vi "LVClass_CorrectionDataManager SetWaveFrontCorrectorPreferences.vi"(0 "CorrectionDataManager in":refnum<class "CorrectionDataManager.lvclass">, 9 "Wavefront Corrector State":T1[](array[typedef]), 11 "error in (no error)":errorcluster) -> (4 "CorrectionDataManager out":refnum<class "CorrectionDataManager.lvclass">, 8 "New data needed":bool, 15 "error out":errorcluster)   [LabVIEW 2020, in "CorrectionDataManager.lvclass"]
doc: "Wavefront corrector actuators preferences setter. The new preferences have to\nbe compliant with the Wavefront corrector specifications (read from\nconfiguration file).\n\n--------------------------------------------------------------------------------\n\n<B>corrdata_managerIn </B> : CorrDataManager object.\n<B>corrdata_managerOut </B> : CorrDataManager object.\n<B>min </B> : WavefrontCorrector preferences : lowest command value.\n<B>max </B> : WavefrontCorrector preferences : highest command value.\n<B>validity </B> : WavefrontCorrector preferences : status.\n<B>fixed_value </B> : WavefrontCorrector preferences : fixed positions.\n<B>ErrorIn </B> : Error\n<B>ErrorOut </B> : Error\n\n--------------------------------------------------------------------------------"
uses:
  CorrectionDataManager.lvclass
  Wavefront Corrector states - ONE.ctl
  CorrectionDataManager.lvclass/CorrectionDataManager.ctl
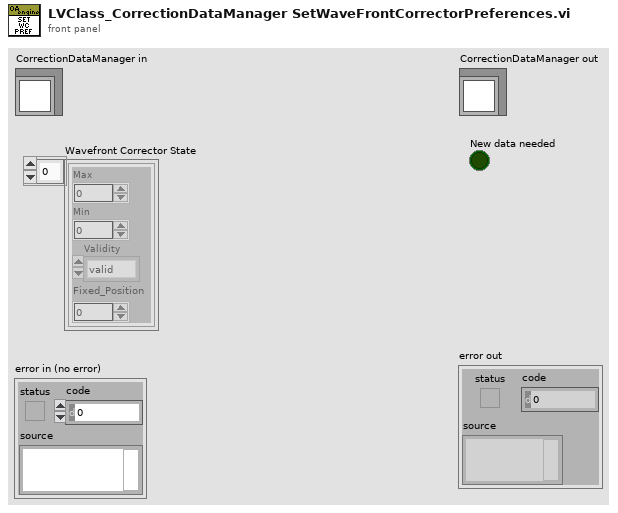
[diagram p1: front panel]
types:
  T1 = typedef "Wavefront Corrector states - ONE.ctl" = cluster{"Max":sgl, "Min":sgl, "Validity":enum16{"valid", "fixed", "invalid"}, "Fixed_Position":sgl}
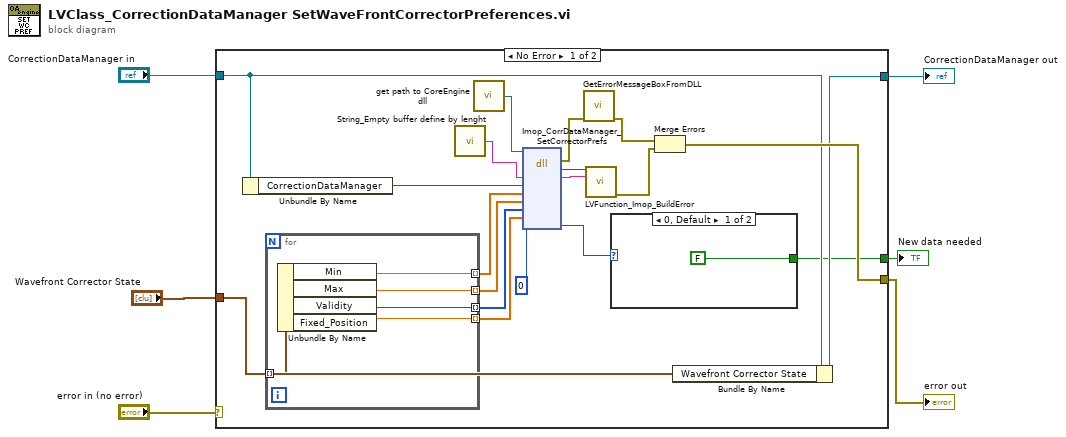
[diagram p0: block diagram]
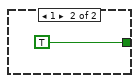
[diagram p2: hidden frame]
diagram:
  n1 = case shown="No Error" "error in (no error)" {
    selector: "error in (no error)" -> [_ w34]
    tunnel: [w23 w34] -> w3
    tunnel: [w11 w33] -> w4
    tunnel: "CorrectionDataManager in" -> [w12 w33]
    tunnel: "Wavefront Corrector State" -> [w10 _]
    tunnel: [w7 _] -> w1
    frame No Error {
      n2 = Unbundle By Name(w12) -> ("CorrectionDataManager"=w13:i32)
      n3 = for {
        tunnel: w10 -> [w32] mode=indexing
        tunnel: [w31] -> w15 mode=indexing
        tunnel: [w30] -> w14 mode=indexing
        tunnel: [w29] -> w17 mode=indexing
        tunnel: [w28] -> w16 mode=indexing
        n4 = Unbundle By Name(w32) -> ("Min"=w31:sgl, "Max"=w30:sgl, "Validity"=w29:enum16{"valid", "fixed", "invalid"}, "Fixed_Position"=w28:sgl)
      }
      n5 = call "String_Empty buffer define by lenght.vi"() -> ("Empty buffer"=w21:string)  [unwired: 1 in]
      n6 = call "get path to CoreEngine dll.vi"() -> ("path to c_interface_vc100.dll"=w22:path)  [unwired: 12 in, 3 out]
      n7 = dll-call lib="D:/soft/HASO_v3/SVN_trunk/ImOpCoreEngine4_LV2011/DLLs/c_interface_vc100.dll" fn="Imop_CorrDataManager_SetCorrectorPrefs"(path in=w22, "message"=w21, "CorrDataManager"=w13, "min"=w15, "max"=w14, "validity"=w17, "fixed_value"=w16, "New data needed"=u8 0) -> (error out=w20:errorcluster, "return type"=w19:i32, "message"=w18:string, "New data needed"=w8:u8)  [unwired: 7 in, 1 out]
      n8 = call "GetErrorMessageBoxFromDLL.vi"("error IN"=w20) -> ("error OUT"=w25:errorcluster)  [unwired: 10 in]
      n9 = call "LVFunction_Imop_BuildError.vi"("code"=w19, "String to Prepend to source (\"\")"=w18) -> ("error out"=w24:errorcluster)  [unwired: 13 in]
      n10 = case shown="0, Default" w8 {
        tunnel: [FALSE TRUE] -> w7
        frame 0, Default {
        }
        frame 1 {
        }
      }
      n11 = Merge Errors(w25, w24) -> (w23:errorcluster)
      n12 = Bundle By Name(cluster=w12, "Wavefront Corrector State"=w10) -> (w11:refnum<class "CorrectionDataManager.lvclass">)
    }
    frame Error {
    }
  }
  "error out" <- w3
  "CorrectionDataManager out" <- w4
  "New data needed" <- w1
